vi "Handle New Client.vi"(8 "error in (no error)":errorcluster, 10 "WS Client":refnum<class "WebSocket Client.lvclass">, 11 "WebSocket Handler in":refnum<class "WebSocket Handler.lvclass">) -> (0 "error out":errorcluster, 3 "WebSocket Handler out":refnum<class "WebSocket Handler.lvclass">)   [LabVIEW 2020, in "HTTP Server.lvlib" / "WebSocket Handler.lvclass"]
uses:
  WebSocket Handler.lvclass/WebSocket Handler.ctl
  WebSocket Handler.lvclass
  WebSocket Manager/WebSocket Manager.lvclass
  WebSocket Client/WebSocket Client.lvclass
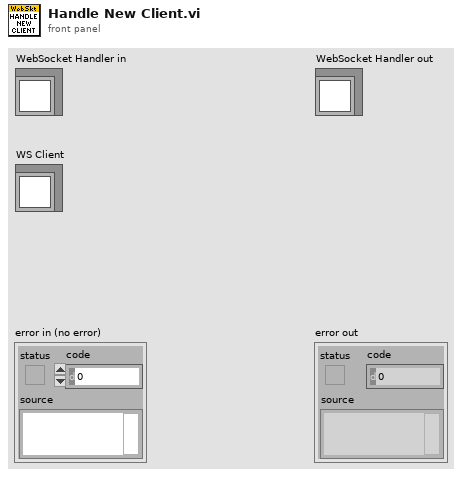
[diagram p1: front panel]
types:
  T1 = typedef "HTTP Server.lvlib/WebSocket Data.ctl" = cluster{"WS Managers":map{string, refnum<class "WebSocket Manager.lvclass">}}
  T2 = map{string, refnum<class "WebSocket Manager.lvclass">}
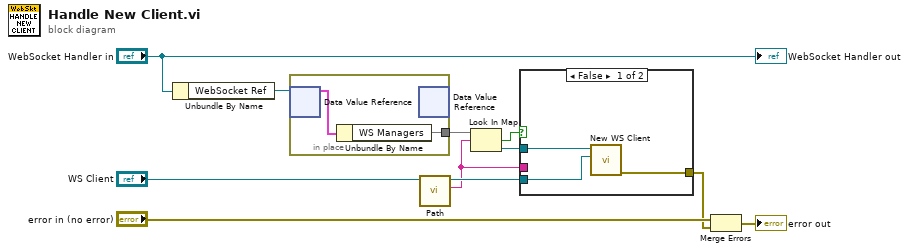
[diagram p0: block diagram]
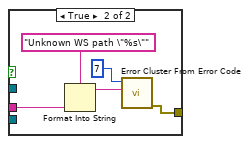
[diagram p2: hidden frame]
diagram:
  n1 = Unbundle By Name("WebSocket Handler in") -> ("WebSocket Ref"=w10:refnum<data-value>)
  n2 = in-place {
    in-place-border: [w12] -> w8
    n3 = in-place-dvr #1(w10) -> (w13:T1)  [unwired: 1 out]
    n4 = Unbundle By Name(w13) -> ("WS Managers"=w12:T2)
    n5 = in-place-dvr #1() -> ()  [unwired: 1 in, 2 out]
  }
  n6 = call "Path.vi"("WebSocket Client in"="WS Client") -> ("Path"=w3:string, "WebSocket Client out"=w4:refnum<class "WebSocket Client.lvclass">)  [unwired: 9 in]
  n7 = Look In Map(map=w8, key=w3) -> (key not found?=w6:bool, value=w5:refnum<class "WebSocket Manager.lvclass">)  [unwired: 1 in]
  n8 = case shown="False" w6 {
    tunnel: w5 -> [w16 _]
    tunnel: w4 -> [w15 _]
    tunnel: [w14 w17] -> w1
    tunnel: w3 -> [_ w19]
    frame False {
      n9 = call-dynamic "New WS Client.vi"("WebSocket Client"=w15, "WebSocket Manager in"=w16) -> ("error out"=w14:errorcluster)  [unwired: 8 in, 1 out]
    }
    frame True {
      n10 = Format Into String(format string="Unknown WS path \"%s\"", w19) -> (resulting string=w18:string)  [unwired: 2 in, 1 out]
      n11 = call <vilib>:"Error Cluster From Error Code.vi"("error message (\"\")"=w18, "error code (0)"=7) -> ("error out"=w17:errorcluster)  [unwired: 7 in]
    }
  }
  n12 = Merge Errors("error in (no error)", w1) -> (→"error out":errorcluster)
  "WebSocket Handler out" <- "WebSocket Handler in"
